vi "Deposit.vi"(8 "error in (no error)":errorcluster, 10 "Amount":dbl, 11 "SimpleExpenseAccount in":refnum<class "SimpleExpenseAccount.lvclass">) -> (0 "error out":errorcluster, 2 "Balance":dbl, 3 "SimpleExpenseAccount out":refnum<class "SimpleExpenseAccount.lvclass">)   [LabVIEW 2020, in "SimpleExpenseAccount.lvclass"]
uses:
  SimpleExpenseAccount.lvclass
  SimpleExpenseAccount.lvclass/SimpleExpenseAccount.ctl
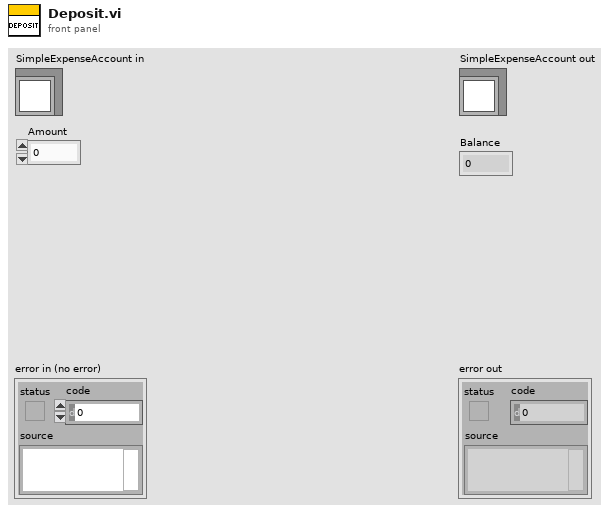
[diagram p1: front panel]
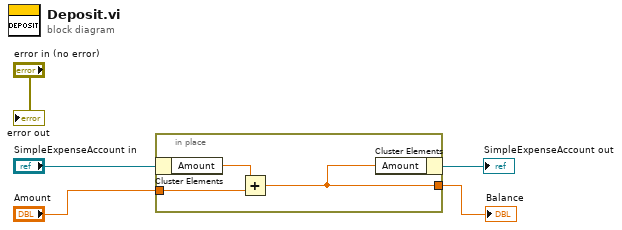
[diagram p0: block diagram]
diagram:
  n1 = in-place {
    in-place-border: "Amount" -> [w7]
    in-place-border: [w6] -> w1
    n2 = in-place-cluster #1("SimpleExpenseAccount in") -> ("Amount"=w8:dbl)
    n3 = Add(x=w8, y=w7) -> (x+y=w6:dbl)
    n4 = in-place-cluster #1("Amount"=w6) -> (→"SimpleExpenseAccount out":refnum<class "SimpleExpenseAccount.lvclass">)
  }
  "Balance" <- w1
  "error out" <- "error in (no error)"
